vi "Waveform_Extract from Start and End Dbl with End point.vi"(8 "Error":errorcluster, 9 "End Time":dbl, 10 "Begin Time":dbl, 11 "Waveform":T1) -> (0 "Error Out":errorcluster, 1 "End Index Out":i32, 2 "Start Index Out":i32, 3 "Waveform Out":T1)   [LabVIEW 2020]
doc: "Retrieves a subset of a waveform at a specified time or index. You must manually select the polymorphic instance you want to use."
uses:
  Universal Controls/Waveform_Data.ctl
  Universal Controls/Read Write Button.ctl
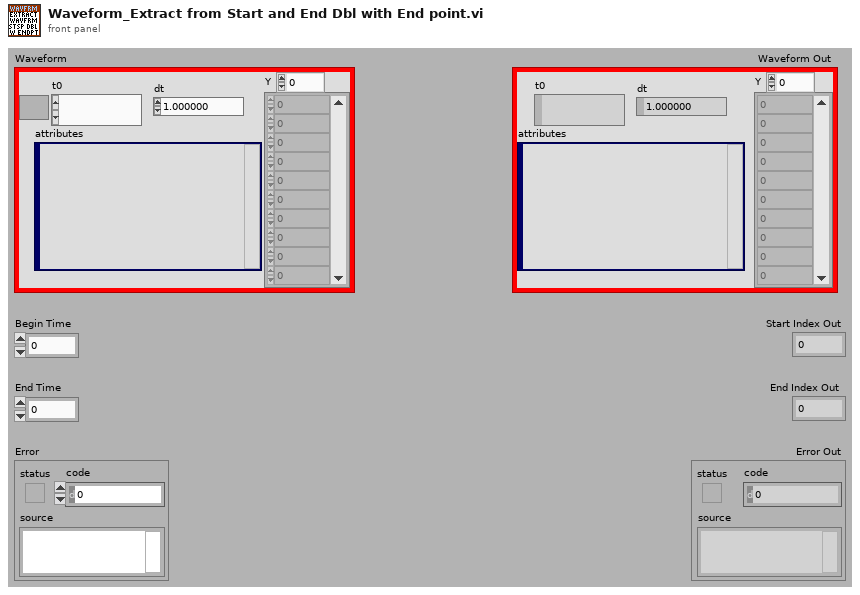
[diagram p1: front panel]
types:
  T1 = typedef "Waveform_Data.ctl" = waveform(dbl)
  T2 = typedef "Read Write Button.ctl" = bool
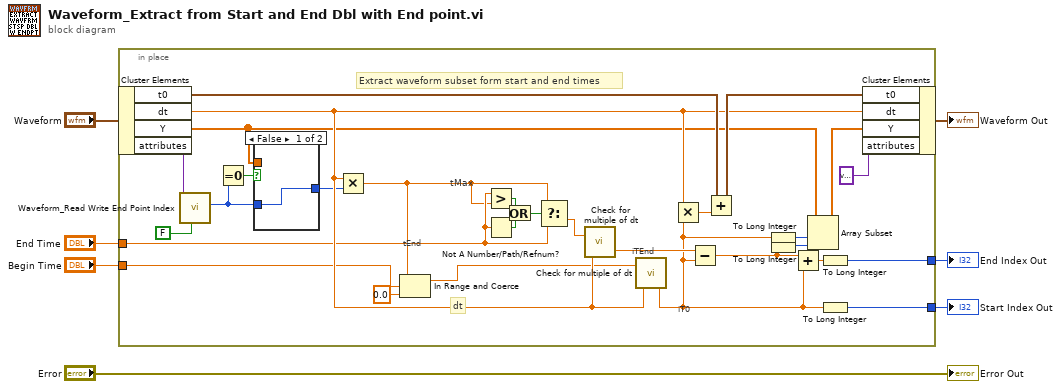
[diagram p0: block diagram]
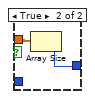
[diagram p2: hidden frame]
diagram:
  n1 = in-place {
    in-place-border: "Begin Time" -> [w16]
    in-place-border: "End Time" -> [w21]
    in-place-border: [w32] -> w5
    in-place-border: [w31] -> w4
    # "Extract waveform subset form start and end times"
    # "dt"
    # "iTEnd"
    # "iT0"
    # "tEnd"
    # "tMax"
    n2 = in-place-cluster #1("Waveform") -> ("t0"=w24:timestamp, "dt"=w22:dbl, "Y"=w8:dbl[], "attributes"=w14:variant)
    n3 = call "Waveform_Read Write End Point Index.vi"("Read(f)\nWrite(t)"=T2 FALSE ("Read(f)\nWrite(t)"), "Waveform Attributes"=w14) -> ("End Point Out"=w10:i32)  [unwired: 6 in, 3 out]
    n4 = Equal To 0?(x=w10) -> (x = 0?=w11:bool)
    n5 = case shown="False" w11 {
      tunnel: w10 -> [w37 _]
      tunnel: [w37 w38] -> w9
      tunnel: w8 -> [_ w39]
      frame False {
      }
      frame True {
        n6 = Array Size(array=w39) -> (size(s)=w38:i32)
      }
    }
    n7 = Multiply(x=w22, y=w9) -> (x*y=w18:dbl)
    n8 = In Range and Coerce(upper limit=w18, x=w16, lower limit=0.0) -> (coerced(x)=w15:dbl)  [unwired: 1 out]
    n9 = Greater?(x=w21, y=w18) -> (0:w36:bool)
    n10 = Not A Number/Path/Refnum?(number/path/refnum=w21) -> (NaN/Path/Refnum?=w35:bool)
    n11 = Or(x=w36, y=w35) -> (x .or. y?=w34:bool)
    n12 = Select(t=w18, s=w34, f=w21) -> (s? t:f=w19:dbl)
    n13 = call <vilib>:"Check for multiple of dt.vi"("dt"=w22, "time"=w19) -> ("iQuotient"=w33:dbl)  [unwired: 1 out]
    n14 = call <vilib>:"Check for multiple of dt.vi"("dt"=w22, "time"=w15) -> ("iQuotient"=w30:dbl)  [unwired: 1 out]
    n15 = Multiply(x=w22, y=w30) -> (x*y=w28:dbl)
    n16 = Subtract(x=w33, y=w30) -> (x-y=w20:dbl)
    n17 = Add(x=w24, y=w28) -> (x+y=w23:timestamp)
    n18 = To Long Integer(number=w30) -> (32bit integer=w26:i32)
    n19 = To Long Integer(number=w20) -> (32bit integer=w27:i32)
    n20 = Add(x=w20, y=w30) -> (x+y=w29:dbl)
    n21 = Array Subset(array=w8, index=w26, length=w27) -> (w25:dbl[])
    n22 = To Long Integer(number=w29) -> (32bit integer=w31:i32)
    n23 = To Long Integer(number=w30) -> (32bit integer=w32:i32)
    n24 = in-place-cluster #1("t0"=w23, "dt"=w22, "Y"=w25, "attributes"=variant) -> (→"Waveform Out":T1)
  }
  "Start Index Out" <- w5
  "End Index Out" <- w4
  "Error Out" <- "Error"
